vi "ex_MakeNamesGeneric.vi"(8 "error in (no error)":errorcluster, 9 "Renamed Controls":string[][](array[string]), 11 "VI refnum":refnum<vi>) -> (0 "error out":errorcluster)   [LabVIEW 2017]
doc: "Changes the names of the controls listed in the Renamed Controls array."
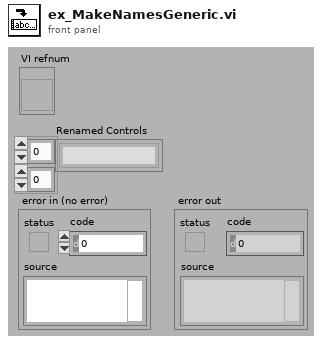
[diagram p1: front panel]
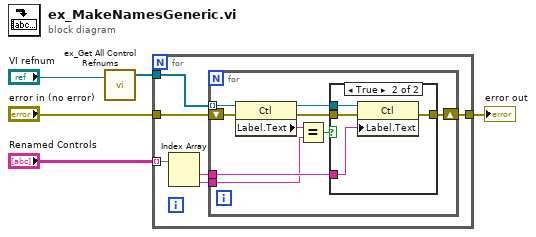
[diagram p0: block diagram]
diagram:
  n1 = call <vilib>:"ex_Get All Control Refnums.vi"("viref Express VI"="VI refnum") -> ("All Controls[]"=w3:refnum<vi>[])  [unwired: 2 in, 1 out]
  n2 = for {
    tunnel: "Renamed Controls" -> [w10] mode=indexing
    tunnel: w3 -> [w7]
    tunnel: [w11] -> w5
    tunnel: "error in (no error)" -> [w8]
    n3 = Index Array(array=w10) -> (element #1=w6:string, element #2=w9:string)  [unwired: 2 in]
    n4 = for {
      tunnel: w7 -> [w20] mode=indexing
      tunnel: w6 -> [w17]
      shift-right: [w14] -> w11
      shift-left: w8 -> [w13]
      tunnel: w9 -> [w12]
      n5 = property class="Ctl"(reference=w20, error in=w13) -> (reference out=w18:refnum<vi>, error out=w15:errorcluster, "Label.Text"=w19:string)
      n6 = Equal?(x=w19, y=w12) -> (x = y?=w16:bool)
      n7 = case shown="True" w16 {
        tunnel: w18 -> [_ w25]
        tunnel: w17 -> [_ w22]
        tunnel: w15 -> [w21 w24]
        tunnel: [w21 w23] -> w14
        frame False {
        }
        frame True {
          n8 = property class="Ctl"(reference=w25, error in=w24, "Label.Text"=w22) -> (error out=w23:errorcluster)  [unwired: 1 out]
        }
      }
    }
  }
  "error out" <- w5
